vi "tlc_Error Module.vi"(7 "Command (Handle Errors":T4=enum."Handle Errors", 8 "error in (no error)":errorcluster, 9 "tlc_Consumer Queue Reference.ctl":T2, 10 "tlc_Display Queue Reference.ctl":T1, 11 "tlc_User Event Reference.ctl":T3) -> (0 "error out":errorcluster, 2 "status":bool)   [LabVIEW 2018]
doc: "Controls access to the Cue data."
uses:
  tlc_Error Module Command Control.ctl
  Controls/tlc_User Event Reference.ctl
  Controls/tlc_Consumer Queue Reference.ctl
  Controls/tlc_Consumer Control.ctl
  Controls/tlc_Functions.ctl
  Controls/tlc_Display Queue Reference.ctl
  Controls/tlc_User Interface Command.ctl
  Controls/tlc_User Interface Data Type.ctl
panel:
  # "Output"
  # "Input"
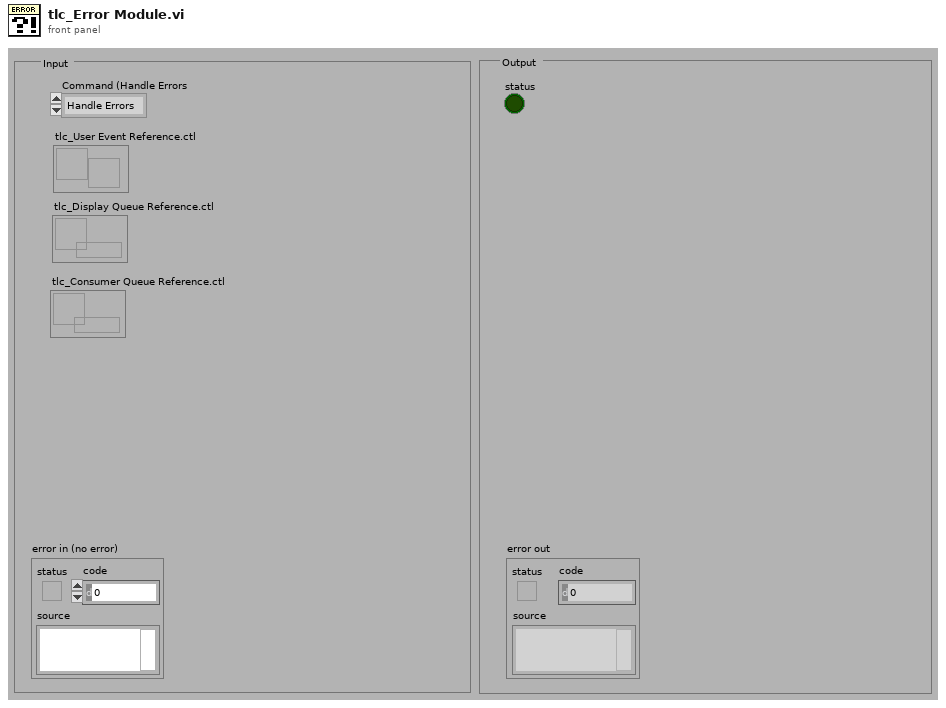
[diagram p1: front panel]
types:
  T1 = typedef "tlc_Display Queue Reference.ctl" = refnum<queue>
  T2 = typedef "tlc_Consumer Queue Reference.ctl" = refnum<queue>
  T3 = typedef "tlc_User Event Reference.ctl" = refnum<user-event>
  T4 = typedef "tlc_Error Module Command Control.ctl" = enum16{"Initialize", "Handle Errors", "Report Errors"}
  T5 = typedef "tlc_Consumer Control.ctl" = cluster{"Command":T6, "Data":variant}
  T6 = typedef "tlc_Functions.ctl" = enum16{"Initialize", "Record", "Load", "Save", "Play", "Move Cue Up", "Move Cue Down", "Select Cue", "Delete", "Stop", "Exit"}
  T7 = typedef "tlc_User Interface Command.ctl" = cluster{"Data Type":T8, "Data":variant}
  T8 = typedef "tlc_User Interface Data Type.ctl" = enum16{"Initialize", "Initialize Front Panel", "Update Front Panel Channels", "Select Cue in Cue List", "Enable/Disable Front Panel Controls", "Update Cue List", "Stop"}
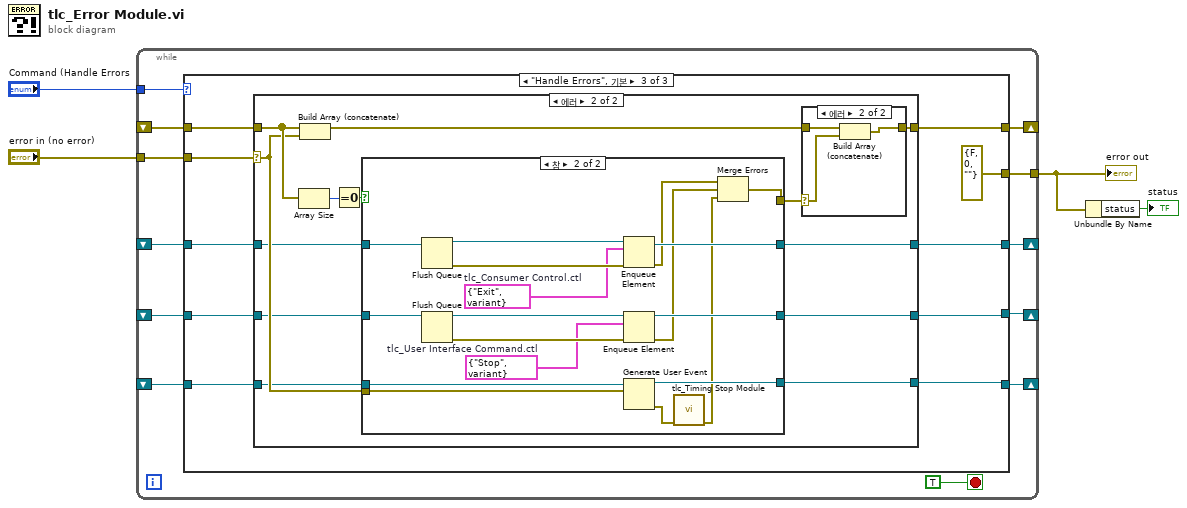
[diagram p0: block diagram]
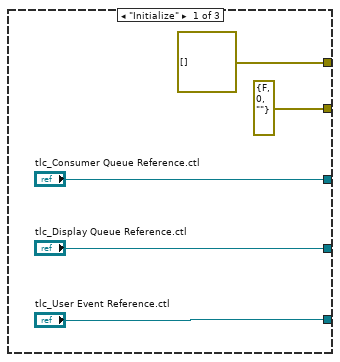
[diagram p2: hidden frame]
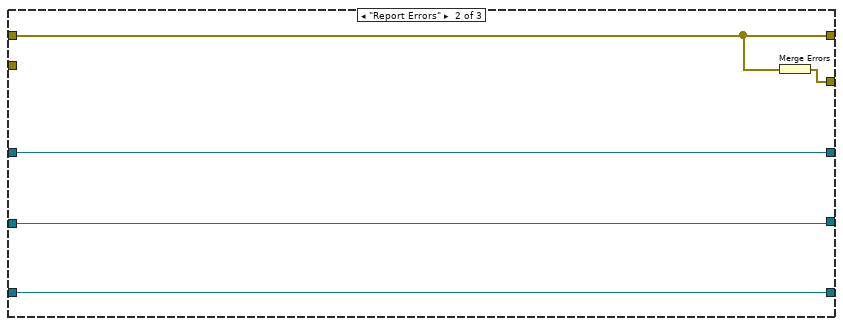
[diagram p3: hidden frame]
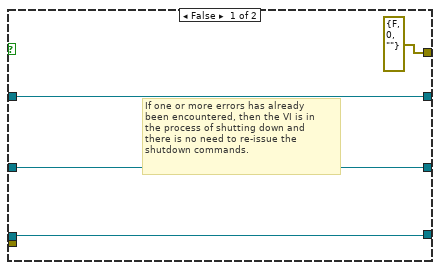
[diagram p6: hidden frame]
diagram:
  n1 = while {
    shift-right: [w12] -> _
    shift-left: _ -> [w14]
    tunnel: "error in (no error)" -> [w15]
    tunnel: "Command (Handle Errors" -> [w13]
    tunnel: [w11] -> w2
    shift-right: [w10] -> _
    shift-left: _ -> [w7]
    shift-right: [w9] -> _
    shift-left: _ -> [w6]
    shift-right: [w8] -> _
    shift-left: _ -> [w5]
    stop <- TRUE stop-if-true
    n2 = case shown="\"Handle Errors\", 기본" w13 {
      tunnel: w15 -> [_ _ w36]
      tunnel: [errorcluster[] [] w25 w34] -> w12
      tunnel: w14 -> [_ w25 w35]
      tunnel: [errorcluster {"status"=FALSE, "code"=0, "source"=""} ("error out") w26 errorcluster {"status"=FALSE, "code"=0, "source"=""} ("error out")] -> w11
      tunnel: ["tlc_Consumer Queue Reference.ctl" w24 w27] -> w10
      tunnel: ["tlc_Display Queue Reference.ctl" w23 w28] -> w9
      tunnel: ["tlc_User Event Reference.ctl" w22 w29] -> w8
      tunnel: w7 -> [_ w24 w32]
      tunnel: w6 -> [_ w23 w31]
      tunnel: w5 -> [_ w22 w30]
      frame "Initialize" {
      }
      frame "Report Errors" {
        n3 = Merge Errors(w25) -> (w26:errorcluster)
      }
      frame "Handle Errors", Default {
        n4 = case shown="에러" w36 {
          selector: w36 -> [_ w47]
          tunnel: [w40 w49] -> w34
          tunnel: w35 -> [w40 w53]
          tunnel: w32 -> [w39 w46]
          tunnel: w31 -> [w38 w45]
          tunnel: w30 -> [w37 w44]
          tunnel: [w37 w43] -> w29
          tunnel: [w38 w42] -> w28
          tunnel: [w39 w41] -> w27
          frame No Error {
          }
          frame Error {
            n5 = Array Size(array=w53) -> (size(s)=w51:i32)
            n6 = Build Array (concatenate)(w53, w47) -> (w50:errorcluster[])
            n7 = Equal To 0?(x=w51) -> (x = 0?=w52:bool)
            n8 = case shown="참" w52 {
              tunnel: [errorcluster {"status"=FALSE, "code"=0, "source"=""} ("error out") w65] -> w48
              tunnel: w47 -> [_ w72]
              tunnel: w46 -> [w60 w79]
              tunnel: w45 -> [w59 w78]
              tunnel: w44 -> [w58 w73]
              tunnel: [w58 w68] -> w43
              tunnel: [w59 w67] -> w42
              tunnel: [w60 w66] -> w41
              frame False {
                # "If one or more errors has already \nbeen encountered, then the VI is in \nthe process of shutting down and \nthere is no need to re-issue the \nshutdown commands."
              }
              frame True {
                w70 = T5 {"Command"=enum."Exit", "Data"=variant}  # tlc_Consumer Control.ctl
                w71 = T7 {"Data Type"=enum."Stop", "Data"=variant}  # tlc_User Interface Command.ctl
                n9 = Flush Queue(queue=w79) -> (queue out=w77:T2, error out=w74:errorcluster)  [unwired: 1 in, 1 out]
                n10 = Flush Queue(queue=w78) -> (queue out=w76:T1, error out=w75:errorcluster)  [unwired: 1 in, 1 out]
                n11 = Enqueue Element(queue=w77, element=w70, error in (no error)=w74) -> (queue out=w66:T2, error out=w64:errorcluster)  [unwired: 1 in, 1 out]
                n12 = Enqueue Element(queue=w76, element=w71, error in (no error)=w75) -> (queue out=w67:T1, error out=w63:errorcluster)  [unwired: 1 in, 1 out]
                n13 = Generate User Event(user event=w73, event data cluster=w72) -> (user event out=w68:T3, error out=w69:errorcluster)  [unwired: 2 in]
                n14 = call "tlc_Timing Stop Module.vi"("error in (no error)"=w69) -> ("error out"=w62:errorcluster)  [unwired: 10 in]
                n15 = Merge Errors(w64, w63, w62) -> (w65:errorcluster)
              }
            }
            n16 = case shown="에러" w48 {
              selector: w48 -> [_ w55]
              tunnel: w50 -> [w54 w57]
              tunnel: [w54 w56] -> w49
              frame No Error {
              }
              frame Error {
                n17 = Build Array (concatenate)(w57, w55) -> (w56:errorcluster[])
              }
            }
          }
        }
      }
    }
  }
  "error out" <- w2
  n18 = Unbundle By Name(w2) -> ("status"=→"status":bool)
